vi "Enable Vent.vi"(7 "Channel (0: Channel A)":u16(ring) items=["Channel A", "Channel B"], 8 "error in (no error)":errorcluster, 10 "Enable Vent (T: On)":bool=TRUE, 11 "BH Druck PACE Series in":refnum<class "BH Druck PACE Series.lvclass">) -> (0 "error out":errorcluster, 3 "BH Druck PACE Series out":refnum<class "BH Druck PACE Series.lvclass">)   [LabVIEW 2022 SP3, in "BH Druck PACE Series.lvclass"]
uses:
  BH Druck PACE Series.lvclass
  BH Druck PACE Series.lvclass/BH Druck PACE Series.ctl
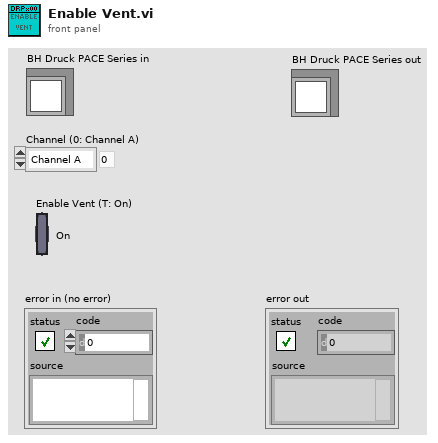
[diagram p1: front panel]
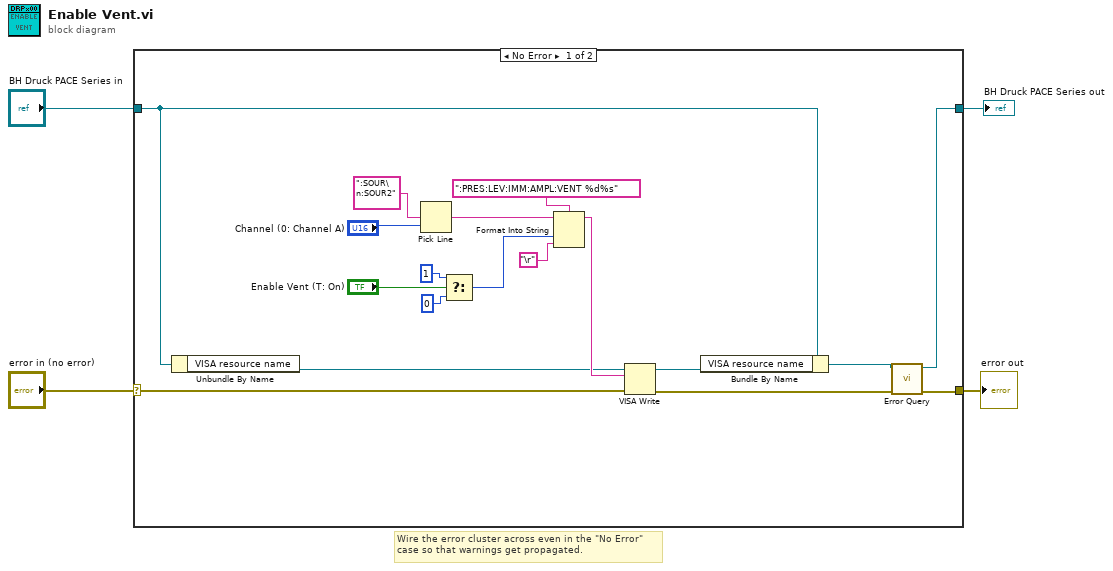
[diagram p0: block diagram]
diagram:
  # "Wire the error cluster across even in the \"No Error\"\ncase so that warnings get propagated."
  n1 = case shown="No Error" "error in (no error)" {
    selector: "error in (no error)" -> [w12 w24]
    tunnel: [w7 w24] -> w3
    tunnel: [w5 w23] -> w1
    tunnel: "BH Druck PACE Series in" -> [w10 w23]
    frame No Error {
      n2 = Unbundle By Name(w10) -> ("VISA resource name"=w11:refnum<visa-resource-name>)
      n3 = Pick Line(multi-line string=":SOUR\n:SOUR2", line index="Channel (0: Channel A)") -> (output string=w20:string)  [unwired: 1 in]
      n4 = Select(t=1, s="Enable Vent (T: On)", f=0) -> (s? t:f=w18:i32)
      n5 = Format Into String(format string=":PRES:LEV:IMM:AMPL:VENT %d%s", initial string=w20, w18, "\r") -> (resulting string=w22:string)  [unwired: 1 in, 1 out]
      n6 = VISA Write(VISA resource name=w11, write buffer=w22, error in (no error)=w12) -> (VISA resource name out=w9:refnum<visa-resource-name>, error out=w8:errorcluster)  [unwired: 1 out]
      n7 = Bundle By Name(cluster=w10, "VISA resource name"=w9) -> (w6:refnum<class "BH Druck PACE Series.lvclass">)
      n8 = call-dynamic "Error Query.vi"("error in (no error)"=w8, "BH Druck PACE Series in"=w6) -> ("error out"=w7:errorcluster, "BH Druck PACE Series out"=w5:refnum<class "BH Druck PACE Series.lvclass">)  [unwired: 8 in]
    }
    frame Error {
    }
  }
  "error out" <- w3
  "BH Druck PACE Series out" <- w1
